vi "Actor Core.vi"(8 "error in":errorcluster, 11 "Measure Object in":refnum<class "PID Controller.lvclass">) -> (0 "error out":errorcluster, 3 "Actor out":refnum<class "Actor.lvclass">)   [LabVIEW 2016, in "PID Controller.lvclass"]
doc: "(<B>Filename</B>: Actor Framework.lvlib:Actor.lvclass:Actor Core.vi)\n\nReceives messages to the actor, reacts to them, and initiates any error handling that may shut the actor down.\n\nDescendant classes may override this VI to append parallel tasks for the actor to complete while it handles messages. Overrides use the Call Parent Method node."
uses:
  PID Controller.lvclass
  C:/github/LabActor/Template Module/Template Module.lvclass
  C:/Program Files/National Instruments/LabVIEW 2016/vi.lib/ActorFramework/Actor/Actor.lvclass
  <vilib>/ActorFramework/Actor/Actor.lvclass
  PID Controller Configuration.ctl
  Template Module/Template Module.lvclass/Template Module.ctl
  <vilib>/ActorFramework/Actor/Actor.lvclass/Actor.ctl
  <vilib>/ActorFramework/Message Enqueuer/Message Enqueuer.lvclass/Message Enqueuer.ctl
  Template Module/Read stop event.vi
  <vilib>/ActorFramework/Message Enqueuer/Init from Existing Queue.vi
  <vilib>/ActorFramework/Message Enqueuer/Enqueue.vi
  Template Module Messages/Configuration Value Changed Msg/Configuration Value Changed Msg.lvclass
  C:/Program Files/National Instruments/LabVIEW 2016/vi.lib/ActorFramework/Message/Message.lvclass
  <vilib>/ActorFramework/Message Priority Queue/Priority Enqueue.vi
  Instrument Actor/Instrument Actor.lvclass
  <vilib>/ActorFramework/Message Enqueuer/Message Enqueuer.lvclass
panel:
  out "Name":string
  in  "Configuration":T1
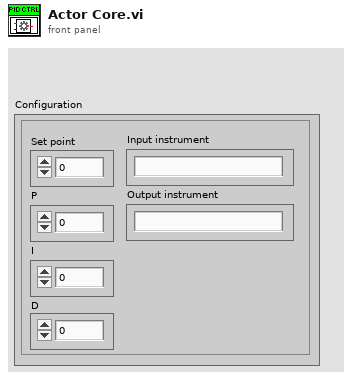
[diagram p1: front panel]
types:
  T1 = typedef "PID Controller Configuration.ctl" = cluster{"P":dbl, "I":dbl, "D":dbl, "Set point":dbl, "Input instrument":string, "Output instrument":string}
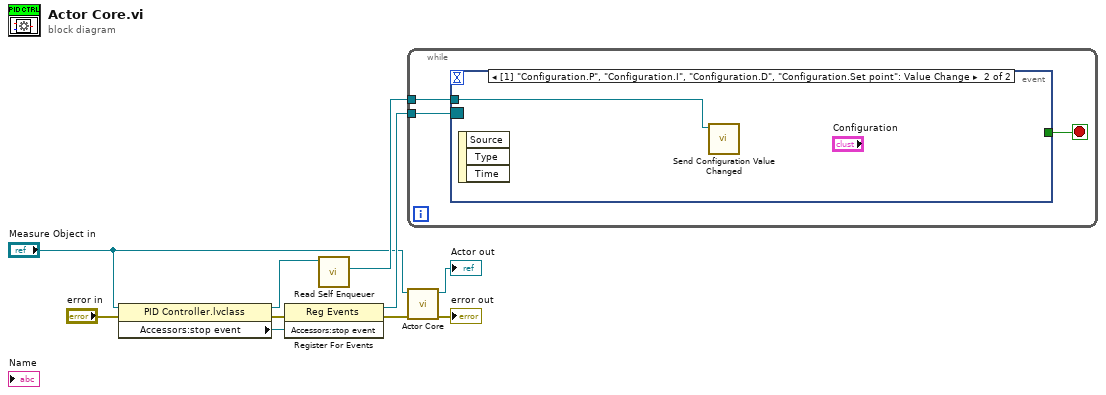
[diagram p0: block diagram]
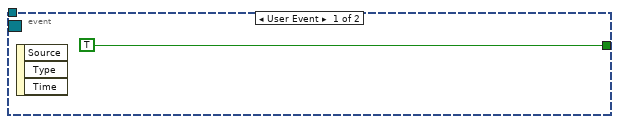
[diagram p2: hidden frame]
diagram:
  n1 = property class="PID Controller.lvclass"(reference="Measure Object in", error in="error in") -> (reference out=w7:refnum<class "PID Controller.lvclass">, error out=w6:errorcluster, "Accessors:stop event"=w4:refnum<user-event>)
  n2 = register-events(error in=w6, w4) -> (reference out=w5:refnum<event-registration>, error out=w1:errorcluster)  [unwired: 1 in]
  n3 = call <vilib>:"Read Self Enqueuer.vi"("Actor"=w7) -> ("Self Enqueuer"=w8:refnum<class "Message Enqueuer.lvclass">)  [unwired: 10 in]
  n4 = while {
    tunnel: w5 -> [w13]
    tunnel: w8 -> [w11]
    stop <- w12 stop-if-true
    n5 = event shown="[1] \"Configuration.P\", \"Configuration.I\", \"Configuration.D\", \"Configuration.Set point\": Value Change" {
      selector: w13 -> [_ _]
      dyn-events: _ -> [_ _]
      timeout: _ -> [_ _]
      tunnel: [TRUE _] -> w12
      tunnel: w11 -> [_ w15]
      event User Event {
        n6 = event-data() -> ()  [unwired: 1 in, 3 out]
      }
      event Value Change {
        n7 = event-data() -> ()  [unwired: 1 in, 3 out]
        n8 = call "Send Configuration Value Changed.vi"("Message Enqueuer"=w15) -> ()  [unwired: 9 in, 2 out]
      }
    }
  }
  n9 = call-parent "Actor Core.vi"("error in"=w1, "Measure Object in"="Measure Object in") -> ("error out"=→"error out":errorcluster, "Actor out"=→"Actor out":refnum<class "Actor.lvclass">)  [unwired: 8 in]
